vi "Set Vi_Button.vi"(8 "error in (no error)":errorcluster, 9 "Open Window":bool, 10 "VI Refnum":refnum<vi>, 11 "Vi_Button in":refnum<class "Vi_Button.lvclass">) -> (0 "error out":errorcluster, 3 "Vi_Button out":refnum<class "Vi_Button.lvclass">)   [LabVIEW 2012, in "Vi_Button.lvclass"]
doc: "An extra mathod to load the vi into the class"
uses:
  Vi_Button.lvclass
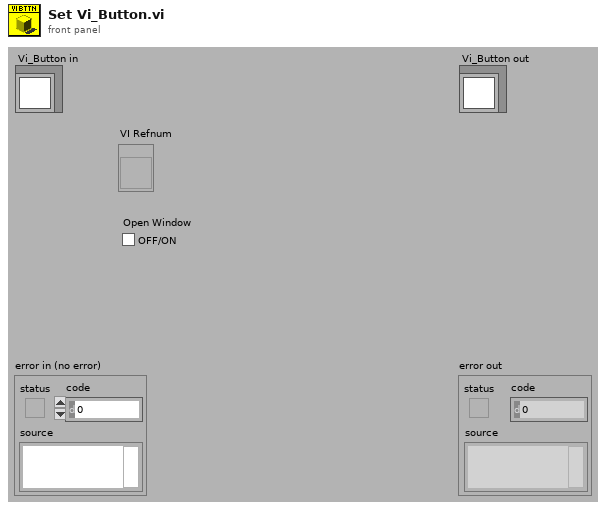
[diagram p1: front panel]
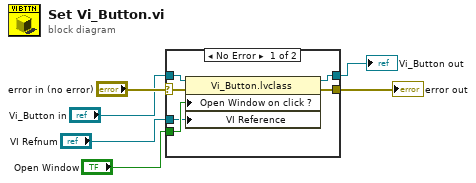
[diagram p0: block diagram]
diagram:
  n1 = case shown="No Error" "error in (no error)" {
    selector: "error in (no error)" -> [w10 w14]
    tunnel: [w9 w14] -> w5
    tunnel: [w11 w13] -> w3
    tunnel: "Vi_Button in" -> [w12 w13]
    tunnel: "VI Refnum" -> [w7 _]
    tunnel: "Open Window" -> [w8 _]
    frame No Error {
      n2 = property class="Vi_Button.lvclass"(reference=w12, error in=w10, "Open Window on click ?"=w8, "VI Reference"=w7) -> (reference out=w11:refnum<class "Vi_Button.lvclass">, error out=w9:errorcluster)
    }
    frame Error {
    }
  }
  "error out" <- w5
  "Vi_Button out" <- w3
